vi "Interface_Dispatch_Process Module.vi"(8 "error in (no error)":errorcluster, 10 "TagBus DVR":refnum<data-value>, 11 "Dispatch_SOC Control in":refnum<class "Dispatch_SOC Control.lvclass">) -> (0 "error out":errorcluster, 2 "TagBus DVR out":refnum<data-value>, 3 "Dispatch_SOC Control out":refnum<class "Dispatch_SOC Control.lvclass">)   [LabVIEW 2015, in "Dispatch_SOC Control.lvclass"]
uses:
  Dispatch_SOC Control.lvclass
  TagBus/TagBus.lvclass
panel:
  out "Module Output":cluster{"EnergyStorage_kW setpoint":dbl}
  in  "Module Dependencies":cluster{"EnergyStorage_kW":dbl}
  in  "Module Parameters":cluster{"SOC Control_Target SOC":dbl}
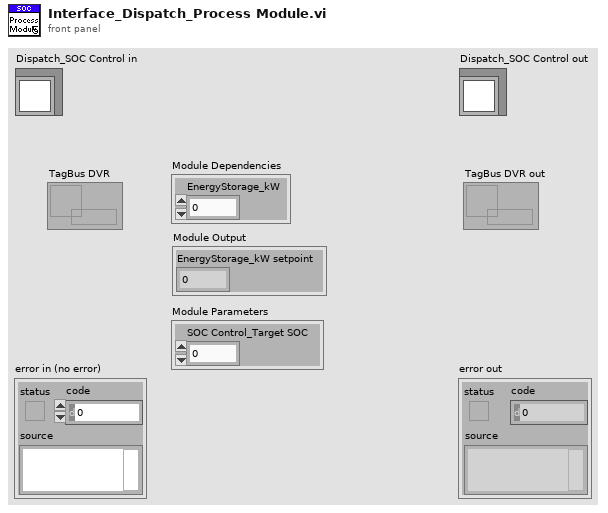
[diagram p1: front panel]
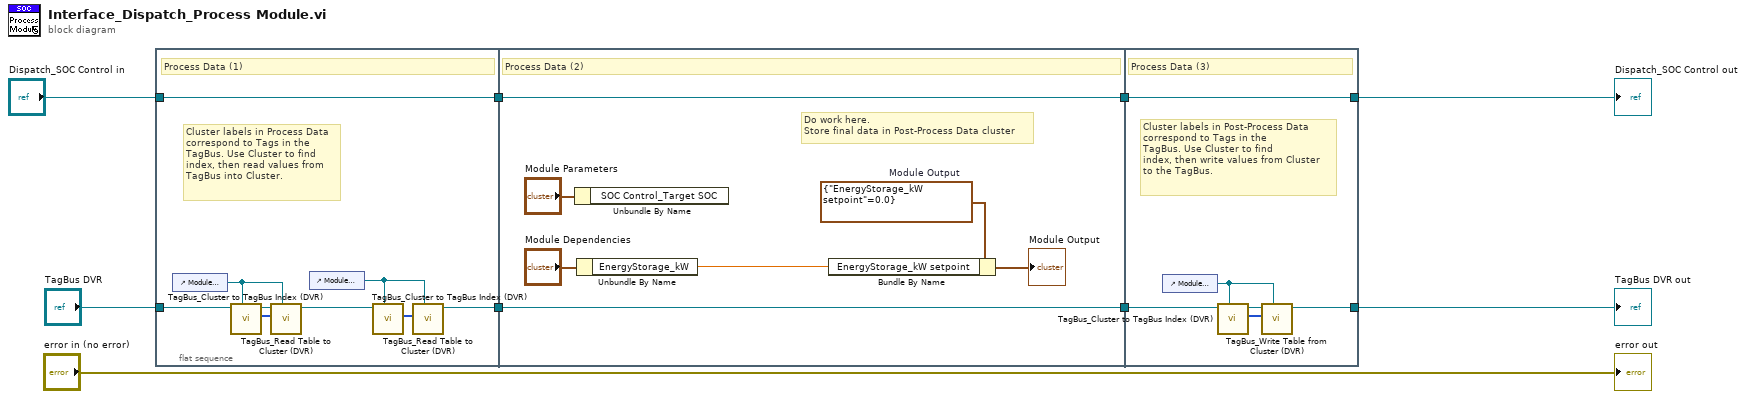
[diagram p0: block diagram]
diagram:
  n1 = flat-sequence {
    tunnel: [w13] -> w9
    tunnel: "Dispatch_SOC Control in" -> [w16]
    tunnel: [w16] -> w5
    tunnel: "TagBus DVR" -> [w10]
    tunnel: w9 -> [w25]
    tunnel: [w25] -> w8
    tunnel: [w23] -> w6
    tunnel: w5 -> [w23]
    tunnel: w8 -> [w31]
    tunnel: w6 -> [w28]
    tunnel: [w28] -> w4
    tunnel: [w26] -> w1
    frame #0 {
      # "Cluster labels in Process Data\ncorrespond to Tags in the\nTagBus. Use Cluster to find\nindex, then read values from\nTagBus into Cluster."
      # "Process Data (1)"
      n2 = control-ref of="Module Parameters"() -> (w12:refnum<vi>)
      n3 = call "TagBus_Cluster to TagBus Index (DVR).vi"("Clust Refnum"=w12, "TagBus DVR"=w10) -> ("Index Array"=w18:i32[], "TagBus DVR out"=w17:refnum<data-value>)  [unwired: 8 in]
      n4 = call "TagBus_Read Table to Cluster (DVR).vi"("Clust Refnum"=w12, "Index Array"=w18, "Data Value Reference in"=w17) -> ("Data Value Reference out"=w14:refnum<data-value>)  [unwired: 8 in]
      n5 = control-ref of="Module Dependencies"() -> (w11:refnum<vi>)
      n6 = call "TagBus_Cluster to TagBus Index (DVR).vi"("Clust Refnum"=w11, "TagBus DVR"=w14) -> ("Index Array"=w15:i32[])  [unwired: 8 in, 1 out]
      n7 = call "TagBus_Read Table to Cluster (DVR).vi"("Clust Refnum"=w11, "Index Array"=w15) -> ("Data Value Reference out"=w13:refnum<data-value>)  [unwired: 9 in]
    }
    frame #1 {
      w24 = cluster{"EnergyStorage_kW setpoint":dbl} {"EnergyStorage_kW setpoint"=0.0}  # Module Output
      # "Do work here.\nStore final data in Post-Process Data cluster"
      # "Process Data (2)"
      n8 = Unbundle By Name("Module Parameters") -> ()  [unwired: 1 out]
      n9 = Unbundle By Name("Module Dependencies") -> ("EnergyStorage_kW"=w19:dbl)
      n10 = Bundle By Name(cluster=w24, "EnergyStorage_kW setpoint"=w19) -> (→"Module Output":cluster{"EnergyStorage_kW setpoint":dbl})
    }
    frame #2 {
      # "Cluster labels in Post-Process Data\ncorrespond to Tags in the\nTagBus. Use Cluster to find\nindex, then write values from Cluster\nto the TagBus."
      # "Process Data (3)"
      n11 = control-ref of="Module Output"() -> (w27:refnum<vi>)
      n12 = call "TagBus_Cluster to TagBus Index (DVR).vi"("Clust Refnum"=w27, "TagBus DVR"=w31) -> ("Index Array"=w30:i32[], "TagBus DVR out"=w29:refnum<data-value>)  [unwired: 8 in]
      n13 = call "TagBus_Write Table from Cluster (DVR).vi"("Clust Refnum"=w27, "Index Array"=w30, "Data Value Reference in"=w29) -> ("Data Value Reference out"=w26:refnum<data-value>)  [unwired: 8 in]
    }
  }
  "error out" <- "error in (no error)"
  "Dispatch_SOC Control out" <- w4
  "TagBus DVR out" <- w1
